vi "Convert String to Numeric.vi"(10 "Channels (A:B:C:D...) (In)":string, 11 "Channel Names (In)":string[](array[string])) -> (2 "Channels (Out)":i32[](array[numeric]), 3 "Channel List (Out)":string[](array[string]))   [LabVIEW 2020]
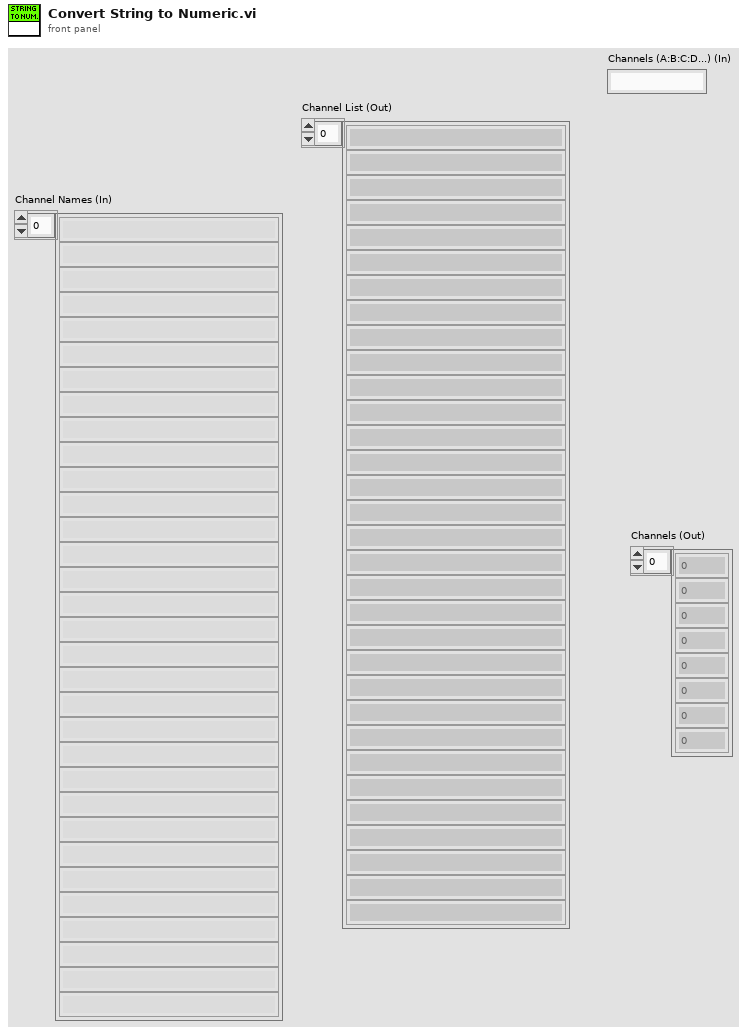
[diagram p1: front panel]
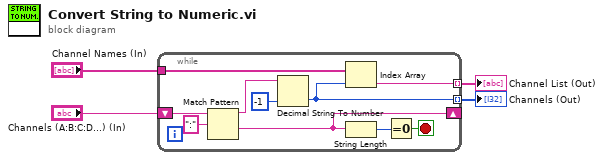
[diagram p0: block diagram]
diagram:
  n1 = while {
    shift-right: [w12] -> _
    shift-left: "Channels (A:B:C:D...) (In)" -> [w14]
    tunnel: "Channel Names (In)" -> [w9]
    tunnel: [w7] -> w2 mode=indexing
    tunnel: [w6] -> w1 mode=indexing
    stop <- w10 stop-if-true
    n2 = Match Pattern(string=w14, regular expression=":") -> (before substring=w5:string, after substring=w12:string)  [unwired: 1 in, 2 out]
    n3 = Decimal String To Number(string=w5, default (0L)=-1 ("default (0 I32)")) -> (number=w6:i32)  [unwired: 1 in, 1 out]
    n4 = Index Array(array=w9, index=w6) -> (element=w7:string)
    n5 = String Length(string=w12) -> (length=w11:i32)
    n6 = Equal To 0?(x=w11) -> (x = 0?=w10:bool)
  }
  "Channel List (Out)" <- w2
  "Channels (Out)" <- w1
